vi "Write Key Ref.vi"(6 "Key Name":string, 7 "Section":string, 8 "error in (no error)":errorcluster, 10 "Section Element":variant, 11 "Refnum in":T1) -> (0 "error out":errorcluster, 3 "Refnum out":T1)   [LabVIEW 2024, in "Generic Config Handling.lvlib"]
doc: "This vi writes a variant to a config file.\n\nIt only accepts very basic datatypes. \n\nIt will accept 1D and 2D arrays.\n\nIf key name is not wired, then it will use the name of the section element."
uses:
  Generic Config Handling.lvlib
  <vilib>/Utility/config.llb/Config Data RefNum.ctl
  <vilib>/Utility/config.llb/Write Key (I32).vi
  <vilib>/Utility/config.llb/Write Key (U32).vi
  <vilib>/Utility/config.llb/Write Key (Double).vi
  <vilib>/Utility/config.llb/Write Key (Boolean).vi
  <vilib>/Utility/config.llb/Write Key (String).vi
  <vilib>/Utility/config.llb/Write Key (Path).vi
  <vilib>/Utility/VariantDataType/VariantType.lvlib
  <vilib>/Utility/config.llb/NI_LVConfig.lvlib
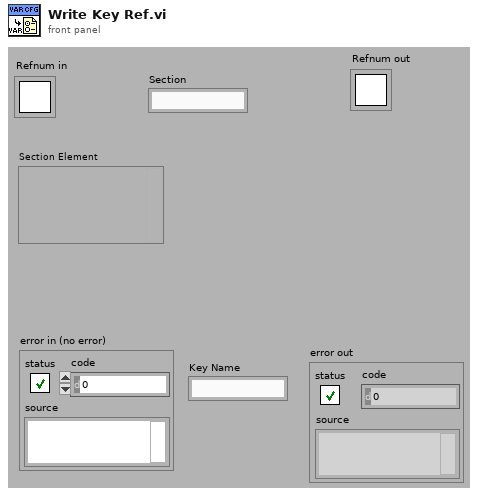
[diagram p1: front panel]
types:
  T1 = typedef "NI_LVConfig.lvlib/Config Data RefNum.ctl" = refnum<k1>
  T2 = typedef "VariantType.lvlib/Type.ctl" = enum8{"Invalid Type", "Void", "I8", "I16", "I32", "I64", "U8", "U16", "U32", "U64", "Single Float", "Double Float", "Extended Float", "Single Complex", "Double Complex", "Extended Complex", "Enum U8", "Enum U16", "Enum U32", "Enum U64", "Single Float With Unit", "Double Float With Unit", "Extended Float With Unit", "Single Complex with Unit", "Double Complex with Unit", "Extended Complex with Unit", "Boolean", "String", "Path", "Picture", "Tag", "Array", "Cluster", "Variant", "LV Variant", "Waveform", "Timestamp", "Digital Waveform", "Digital Data", "ExpressData", "Refnum", "External Data", "VI", "Poly VI", "LabVIEW Class Instance", "Fixed Point"}
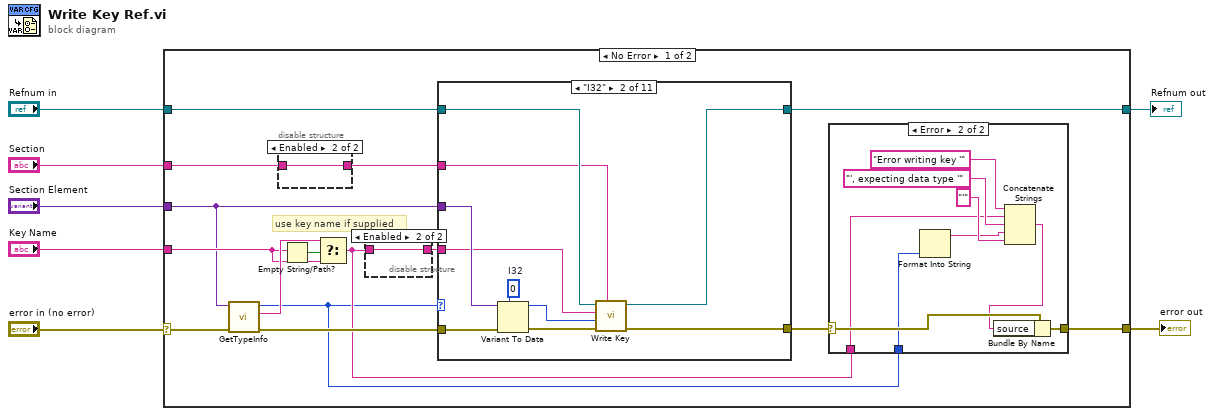
[diagram p0: block diagram]
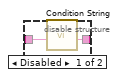
[diagram p2: hidden frame]
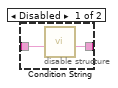
[diagram p3: hidden frame]
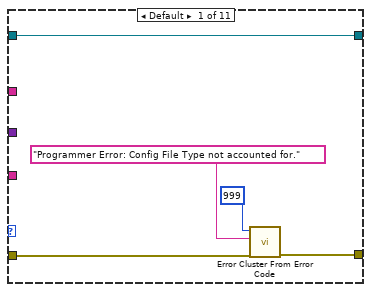
[diagram p5: hidden frame]
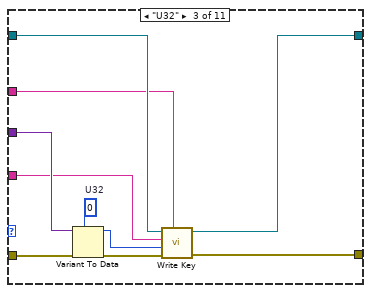
[diagram p6: hidden frame]
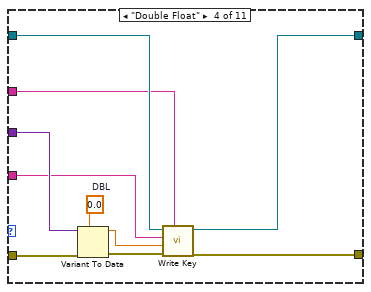
[diagram p7: hidden frame]
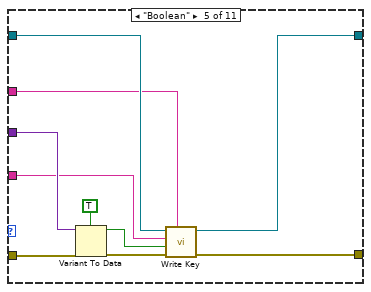
[diagram p8: hidden frame]
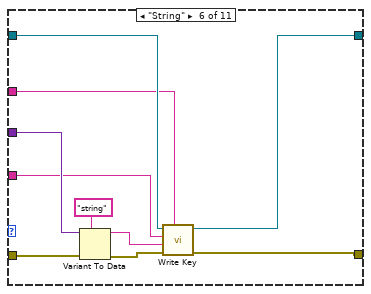
[diagram p9: hidden frame]
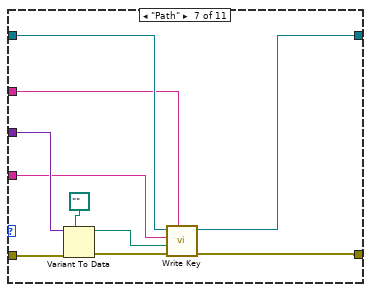
[diagram p10: hidden frame]
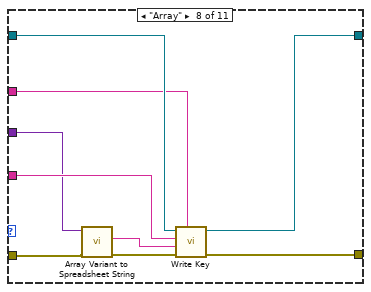
[diagram p11: hidden frame]
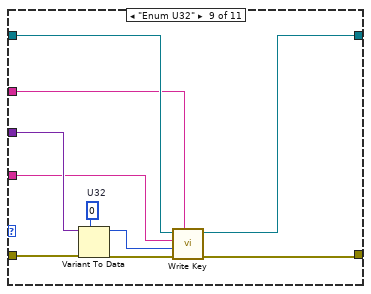
[diagram p12: hidden frame]
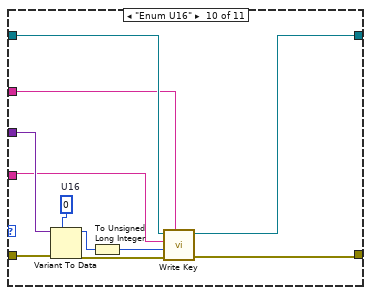
[diagram p13: hidden frame]
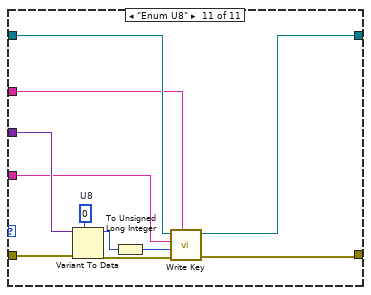
[diagram p14: hidden frame]
diagram:
  n1 = case shown="No Error" "error in (no error)" {
    selector: "error in (no error)" -> [w12 w145]
    tunnel: "Key Name" -> [w20 _]
    tunnel: [w10 w145] -> w6
    tunnel: "Section Element" -> [w19 _]
    tunnel: "Refnum in" -> [w18 w146]
    tunnel: [w17 w146] -> w3
    tunnel: "Section" -> [w16 _]
    frame No Error {
      # "use key name if supplied"
      n2 = call <vilib>:"GetTypeInfo.vi"("error in (no error)"=w12, "Variant"=w19) -> ("error out"=w13:errorcluster, "Name"=w21:string, "Type Enum"=w8:T2)  [unwired: 5 in, 2 out]
      n3 = disable-structure shown="Enabled" {
        disable-tunnel: w16 -> [w27 w28]
        disable-tunnel: [w26 w28] -> w15
        frame Disabled {
          n4 = call "Condition String.vi"("input string"=w27) -> ("result string"=w26:string)  [unwired: 9 in, 1 out]
        }
        frame Enabled {
        }
      }
      n5 = Empty String/Path?(string/path=w20) -> (empty?=w22:bool)
      n6 = Select(t=w21, s=w22, f=w20) -> (s? t:f=w9:string)
      n7 = disable-structure shown="Enabled" {
        disable-tunnel: [w24 w25] -> w14
        disable-tunnel: w9 -> [w23 w25]
        frame Disabled {
          n8 = call "Condition String.vi"("input string"=w23) -> ("result string"=w24:string)  [unwired: 9 in, 1 out]
        }
        frame Enabled {
        }
      }
      n9 = case shown="\"I32\"" w8 {
        tunnel: w13 -> [w41 w47 w59 w67 w77 w88 w99 w105 w117 w128 w139]
        tunnel: w14 -> [_ w44 w56 w64 w74 w85 w96 w108 w114 w125 w136]
        tunnel: [w40 w48 w60 w68 w78 w89 w100 w112 w118 w129 w140] -> w11
        tunnel: w19 -> [_ w53 w63 w73 w83 w93 w103 w107 w122 w133 w144]
        tunnel: w18 -> [w39 w50 w62 w70 w80 w91 w102 w110 w120 w131 w142]
        tunnel: [w39 w49 w61 w69 w79 w90 w101 w111 w119 w130 w141] -> w17
        tunnel: w15 -> [_ w45 w57 w65 w75 w86 w97 w109 w115 w126 w137]
        frame Default {
          n10 = call <vilib>:"Error Cluster From Error Code.vi"("error in (no error)"=w41, "error message (\"\")"="Programmer Error: Config File Type not accounted for." ("error message (\"\")"), "error code (0)"=999) -> ("error out"=w40:errorcluster)  [unwired: 6 in]
        }
        frame "I32" {
          w52 = 0  # I32
          n11 = Variant To Data(error in=w47, type=w52, Variant=w53) -> (data=w51:i32, error out=w46:errorcluster)
          n12 = call-poly <vilib>:"Write Key.vi"("section"=w45, "error in (no error)"=w46, "value"=w51, "key"=w44, "refnum"=w50) -> ("error out"=w48:errorcluster, "refnum out"=w49:T1)  [unwired: 4 in, 1 out]
        }
        frame "U32" {
          w55 = u32 0  # U32
          n13 = Variant To Data(error in=w59, type=w55, Variant=w63) -> (data=w54:u32, error out=w58:errorcluster)
          n14 = call-poly <vilib>:"Write Key.vi"("section"=w57, "error in (no error)"=w58, "value"=w54, "key"=w56, "refnum"=w62) -> ("error out"=w60:errorcluster, "refnum out"=w61:T1)  [unwired: 4 in, 1 out]
        }
        frame "Double Float" {
          w72 = 0.0  # DBL
          n15 = Variant To Data(error in=w67, type=w72, Variant=w73) -> (data=w71:dbl, error out=w66:errorcluster)
          n16 = call-poly <vilib>:"Write Key.vi"("section"=w65, "error in (no error)"=w66, "value"=w71, "key"=w64, "refnum"=w70) -> ("error out"=w68:errorcluster, "refnum out"=w69:T1)  [unwired: 4 in, 1 out]
        }
        frame "Boolean" {
          n17 = Variant To Data(error in=w77, type=TRUE, Variant=w83) -> (data=w81:bool, error out=w76:errorcluster)
          n18 = call-poly <vilib>:"Write Key.vi"("section"=w75, "error in (no error)"=w76, "value"=w81, "key"=w74, "refnum"=w80) -> ("error out"=w78:errorcluster, "refnum out"=w79:T1)  [unwired: 4 in, 1 out]
        }
        frame "String" {
          n19 = Variant To Data(error in=w88, type="string", Variant=w93) -> (data=w92:string, error out=w87:errorcluster)
          n20 = call-poly <vilib>:"Write Key.vi"("section"=w86, "error in (no error)"=w87, "value"=w92, "key"=w85, "refnum"=w91) -> ("error out"=w89:errorcluster, "refnum out"=w90:T1)  [unwired: 4 in, 1 out]
        }
        frame "Path" {
          n21 = Variant To Data(error in=w99, type=path "", Variant=w103) -> (data=w94:path, error out=w98:errorcluster)
          n22 = call-poly <vilib>:"Write Key.vi"("section"=w97, "error in (no error)"=w98, "value"=w94, "key"=w96, "refnum"=w102) -> ("error out"=w100:errorcluster, "refnum out"=w101:T1)  [unwired: 4 in, 1 out]
        }
        frame "Array" {
          n23 = call "Array Variant to Spreadsheet String.vi"("error in (no error)"=w105, "Array Variant"=w107) -> ("error out"=w106:errorcluster, "spreadsheet string"=w104:string)  [unwired: 7 in, 1 out]
          n24 = call-poly <vilib>:"Write Key.vi"("section"=w109, "error in (no error)"=w106, "value"=w104, "key"=w108, "refnum"=w110) -> ("error out"=w112:errorcluster, "refnum out"=w111:T1)  [unwired: 4 in, 1 out]
        }
        frame "Enum U32" {
          w113 = u32 0  # U32
          n25 = Variant To Data(error in=w117, type=w113, Variant=w122) -> (data=w121:u32, error out=w116:errorcluster)
          n26 = call-poly <vilib>:"Write Key.vi"("section"=w115, "error in (no error)"=w116, "value"=w121, "key"=w114, "refnum"=w120) -> ("error out"=w118:errorcluster, "refnum out"=w119:T1)  [unwired: 4 in, 1 out]
        }
        frame "Enum U16" {
          w124 = u16 0  # U16
          n27 = Variant To Data(error in=w128, type=w124, Variant=w133) -> (data=w132:u16, error out=w127:errorcluster)
          n28 = To Unsigned Long Integer(number=w132) -> (unsigned 32bit integer=w123:u32)
          n29 = call-poly <vilib>:"Write Key.vi"("section"=w126, "error in (no error)"=w127, "value"=w123, "key"=w125, "refnum"=w131) -> ("error out"=w129:errorcluster, "refnum out"=w130:T1)  [unwired: 4 in, 1 out]
        }
        frame "Enum U8" {
          w135 = u16 0  # U8
          n30 = Variant To Data(error in=w139, type=w135, Variant=w144) -> (data=w143:u16, error out=w138:errorcluster)
          n31 = To Unsigned Long Integer(number=w143) -> (unsigned 32bit integer=w134:u32)
          n32 = call-poly <vilib>:"Write Key.vi"("section"=w137, "error in (no error)"=w138, "value"=w134, "key"=w136, "refnum"=w142) -> ("error out"=w140:errorcluster, "refnum out"=w141:T1)  [unwired: 4 in, 1 out]
        }
      }
      n33 = case shown="Error" w11 {
        selector: w11 -> [w29 w34]
        tunnel: [w29 w35] -> w10
        tunnel: w9 -> [_ w33]
        tunnel: w8 -> [_ w32]
        frame No Error {
        }
        frame Error {
          n34 = Format Into String(w32) -> (resulting string=w31:string)  [unwired: 3 in, 1 out]
          n35 = Concatenate Strings("Error writing key '" ("string"), w33, "', expecting data type '" ("string"), w31, "'" ("string")) -> (w30:string)
          n36 = Bundle By Name(cluster=w34, "source"=w30) -> (w35:errorcluster)
        }
      }
    }
    frame Error {
    }
  }
  "Refnum out" <- w3
  "error out" <- w6
